vi "Recovery File -- Constant.vi"() -> (2 "Recovery File Path":path)   [LabVIEW 2021]
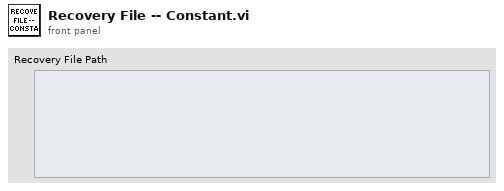
[diagram p1: front panel]
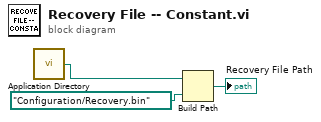
[diagram p0: block diagram]
diagram:
  n1 = call <vilib>:"Application Directory.vi"() -> ("Application Directory"=w3:path)
  n2 = Build Path(base path=w3, name or relative path=path "Configuration/Recovery.bin") -> (appended path=→"Recovery File Path":path)
